vi "Actor Core.vi"(8 "error in":errorcluster, 11 "Console Logger in":refnum<class "Console Logger.lvclass">) -> (0 "error out":errorcluster, 3 "Actor out":refnum<class "Actor.lvclass">)   [LabVIEW 2020, in "Logging.lvlib" / "Console Logger.lvclass"]
doc: "(<B>Filename</B>: Actor Framework.lvlib:Actor.lvclass:Actor Core.vi)\n\nReceives messages to the actor, reacts to them, and initiates any error handling that may shut the actor down.\n\nDescendant classes may override this VI to append parallel tasks for the actor to complete while it handles messages. Overrides use the Call Parent Class Method node."
uses:
  Console Logger.lvclass
  C:/Program Files (x86)/National Instruments/LabVIEW 2020/vi.lib/ActorFramework/Actor/Actor.lvclass
  <vilib>/ActorFramework/Actor/Actor.lvclass
  <vilib>/ActorFramework/Actor/Actor.lvclass/Actor.ctl
  <vilib>/ActorFramework/Message Enqueuer/Message Enqueuer.lvclass/Message Enqueuer.ctl
  <vilib>/ActorFramework/Message Enqueuer/Init from Existing Queue.vi
  <vilib>/ActorFramework/Message Enqueuer/Enqueue.vi
  <vilib>/ActorFramework/Stop Msg/Stop Msg.lvclass
  C:/Program Files (x86)/National Instruments/LabVIEW 2020/vi.lib/ActorFramework/Message/Message.lvclass
  <vilib>/ActorFramework/Message Priority Queue/Priority Enqueue.vi
  <vilib>/ActorFramework/Message Enqueuer/Message Enqueuer.lvclass
  Generic Logger/Generic Logger.lvclass
panel:
  out "Message":string
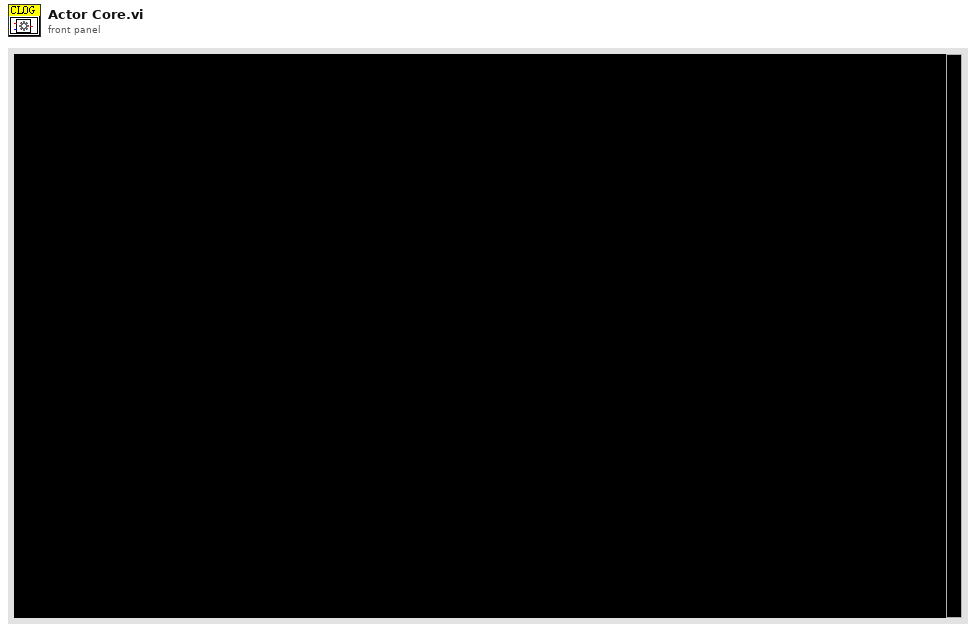
[diagram p1: front panel]
types:
  T1 = enum32{"Invalid", "Standard", "Closed", "Hidden", "Minimized", "Maximized"}
  T2 = cluster{"Stop event":refnum<user-event>, "Log Event":refnum<user-event>}
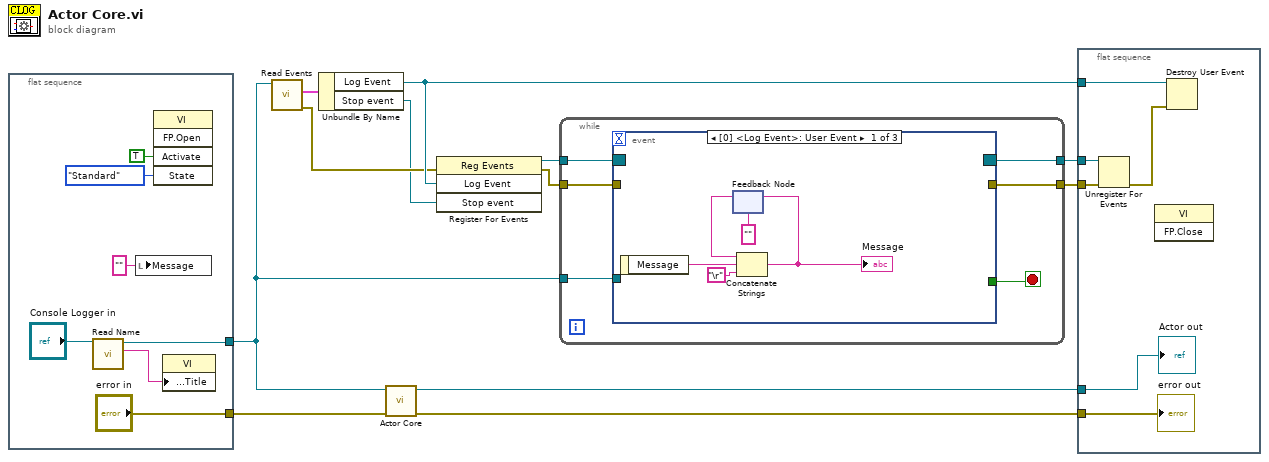
[diagram p0: block diagram]
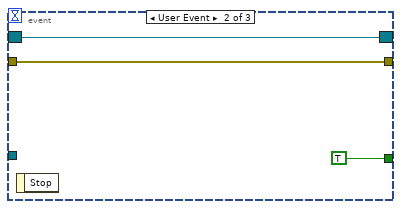
[diagram p2: hidden frame]
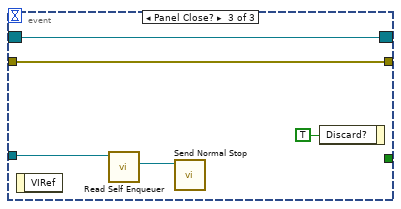
[diagram p3: hidden frame]
diagram:
  n1 = flat-sequence {
    tunnel: ["error in"] -> w10
    tunnel: [w15] -> w1
    frame #0 {
      n2 = call-dynamic "Read Name.vi"("Logger in"="Console Logger in") -> ("Name"=w14:string, "Logger out"=w15:refnum<class "Console Logger.lvclass">)  [unwired: 8 in, 1 out]
      n3 = local write "Message"("" ("Message")) -> ()
      n4 = invoke class="VI" method="FP.Open"("Activate"=TRUE ("Activate?"), "State"=T1."Standard") -> ()  [unwired: 3 in, 5 out]
      n5 = property class="VI"("Front Panel.Title"=w14) -> ()  [unwired: 2 in, 2 out]
    }
  }
  n6 = call-dynamic "Read Events.vi"("Logger in"=w1) -> ("error out"=w3:errorcluster, "Events"=w5:T2)  [unwired: 8 in, 1 out]
  n7 = Unbundle By Name(w5) -> ("Log Event"=w4:refnum<user-event>, "Stop event"=w2:refnum<user-event>)
  n8 = call-parent "Actor Core.vi"("error in"=w10, "Actor in"=w1) -> ("error out"=w12:errorcluster, "Actor out"=w11:refnum<class "Actor.lvclass">)  [unwired: 8 in]
  n9 = register-events(error in=w3, w4, w2) -> (reference out=w9:refnum<event-registration>, error out=w8:errorcluster)  [unwired: 1 in]
  n10 = while {
    tunnel: w9 -> [w25]
    tunnel: w8 -> [w24]
    tunnel: [w22] -> w7
    tunnel: [w21] -> w6
    tunnel: w1 -> [w20]
    stop <- w23 stop-if-true
    n11 = event shown="[0] <Log Event>: User Event" {
      selector: w25 -> [_ w32 w35]
      dyn-events: [_ w32 w35] -> w22
      timeout: _ -> [_ _ _]
      tunnel: w24 -> [_ w31 w34]
      tunnel: [_ TRUE _] -> w23
      tunnel: [_ w31 w34] -> w21
      tunnel: w20 -> [_ _ w36]
      event User Event {
        n12 = event-data() -> ("Message"=w27:string)  [unwired: 1 in]
        n13 = feedback #1("") -> (w28:string)
        n14 = Concatenate Strings(w28, w27, "\r") -> (w29:string)
        "Message" <- w29
        n15 = feedback-in #1(w29) -> ()
      }
      event User Event {
        n16 = event-data() -> ()  [unwired: 1 in, 1 out]
      }
      event Panel Close? {
        n17 = event-data() -> ()  [unwired: 1 in, 1 out]
        n18 = call <vilib>:"Read Self Enqueuer.vi"("Actor"=w36) -> ("Self Enqueuer"=w37:refnum<class "Message Enqueuer.lvclass">)  [unwired: 10 in]
        n19 = call <vilib>:"Send Normal Stop.vi"("Message Enqueuer"=w37) -> ()  [unwired: 10 in, 1 out]
        n20 = event-data("Discard?"=TRUE) -> ()  [unwired: 1 in, 1 out]
      }
    }
  }
  n21 = flat-sequence {
    tunnel: w12 -> [w44]
    tunnel: w11 -> [w39]
    tunnel: w7 -> [w43]
    tunnel: w6 -> [w42]
    tunnel: w4 -> [w40]
    frame #0 {
      n22 = Unregister For Events(event registration refnum=w43, error in=w42) -> (error out=w41:errorcluster)
      n23 = invoke class="VI" method="FP.Close"() -> ()  [unwired: 3 in, 3 out]
      n24 = Destroy User Event(user event=w40, error in=w41) -> ()  [unwired: 1 out]
      "error out" <- w44
      "Actor out" <- w39
    }
  }
